vi "Tosca-Read DI.vi"(0 "Task in":refnum<k21>, 7 "Bits":i32[](array[numeric]), 11 "error in (no error)":errorcluster) -> (4 "Task out":refnum<k21>, 8 "data":bool[](array[boolean]), 15 "error out":errorcluster)   [LabVIEW 2020]
uses:
  <vilib>/DAQmx/read.llb/DAQmx Read (Digital 1D Bool NChan 1Samp 1Line).vi
  <vilib>/DAQmx/miscellaneous.llb/DAQmx Fill In Error Info.vi
  epl-vi-lib/PXI DAQ VIs/TDT VIs/TDT-Globals.vi
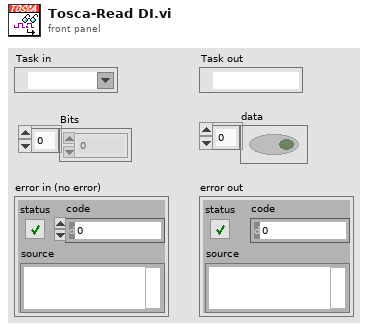
[diagram p1: front panel]
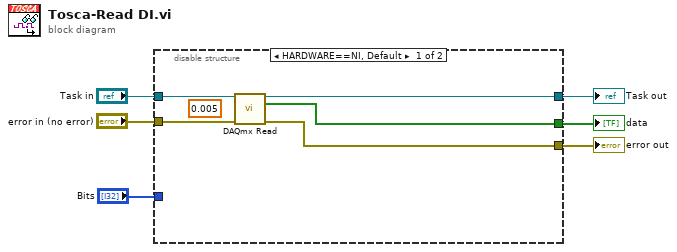
[diagram p0: block diagram]
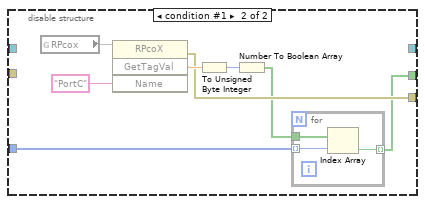
[diagram p2: hidden frame]
diagram:
  n1 = disable-structure shown="HARDWARE==NI, Default" {
    disable-tunnel: [w11 w12] -> w6
    disable-tunnel: [w10 _] -> w5
    disable-tunnel: "error in (no error)" -> [w9 _]
    disable-tunnel: "Task in" -> [w8 _]
    disable-tunnel: [w7 w15] -> w2
    disable-tunnel: "Bits" -> [_ w13]
    frame condition #0 (active) {
      (unwired) 0.005 ("timeout")
      n2 = call-poly <vilib>:"DAQmx Read.vi"("task/channels in"=w8, "error in"=w9) -> ("task out"=w10:refnum<k21>, "data"=w11:bool[], "error out"=w7:errorcluster)  [unwired: 11 in]
    }
    frame condition #1 {
      n3 = global read "TDT-Globals.vi" "RPcox"() -> (w18)
      n4 = invoke class="RPcoX" method="GetTagVal"(reference=w18, "Name"="PortC") -> (error out=w15:errorcluster, "GetTagVal"=w17:sgl)  [unwired: 2 in, 2 out]
      n5 = To Unsigned Byte Integer(number=w17) -> (unsigned 8bit integer=w16:u8)
      n6 = Number To Boolean Array(number=w16) -> (Boolean array=w14:bool[])
      n7 = for {
        tunnel: w14 -> [w22]
        tunnel: w13 -> [w21] mode=indexing
        tunnel: [w20] -> w12 mode=indexing
        n8 = Index Array(array=w22, index=w21) -> (element=w20:bool)
      }
    }
  }
  "data" <- w6
  "Task out" <- w5
  "error out" <- w2
